vi "Execute.vi"(8 "error in (no error)":errorcluster, 9 "Parameters":map{string, variant}(c390), 10 "Query":string, 11 "Sqlite Database Manager in":refnum<class "Sqlite Database Manager.lvclass">) -> (0 "error out":errorcluster, 3 "Sqlite Database Manager out":refnum<class "Sqlite Database Manager.lvclass">)   [LabVIEW 2019, in "HierDAL Library.lvlib" / "Database.lvlib" / "Sqlite Database Manager.lvclass"]
uses:
  Sqlite Database Manager.lvclass
  Sqlite Database Manager.lvclass/Sqlite Database Manager.ctl
  System.Data.SQLite
  <vilib>/Utility/Data Type/NI_Data Type.lvlib
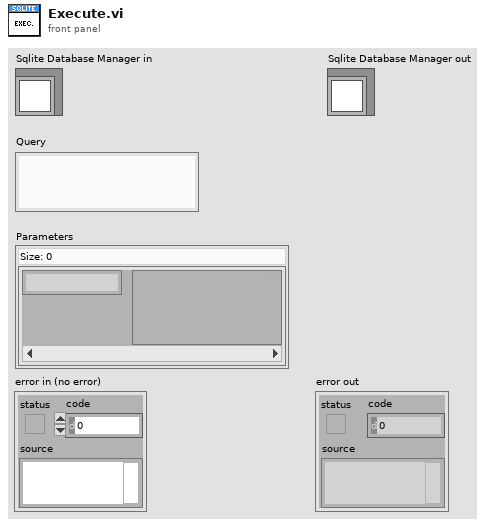
[diagram p1: front panel]
types:
  T1 = typedef "NI_Data Type.lvlib/Data Type.ctl" = enum8{"Invalid Type", "Void", "I8", "I16", "I32", "I64", "U8", "U16", "U32", "U64", "Single Float", "Double Float", "Extended Float", "Single Complex", "Double Complex", "Extended Complex", "Enum U8", "Enum U16", "Enum U32", "Enum U64", "Single Float With Unit", "Double Float With Unit", "Extended Float With Unit", "Single Complex with Unit", "Double Complex with Unit", "Extended Complex with Unit", "Boolean", "String", "Path", "Picture", "Tag", "Array", "Cluster", "Variant", "LV Variant", "Waveform", "Timestamp", "Digital Waveform", "Digital Data", "ExpressData", "Refnum", "External Data", "VI", "Poly VI", "LabVIEW Class Instance", "Fixed Point", "Set Collection", "Map Collection"}
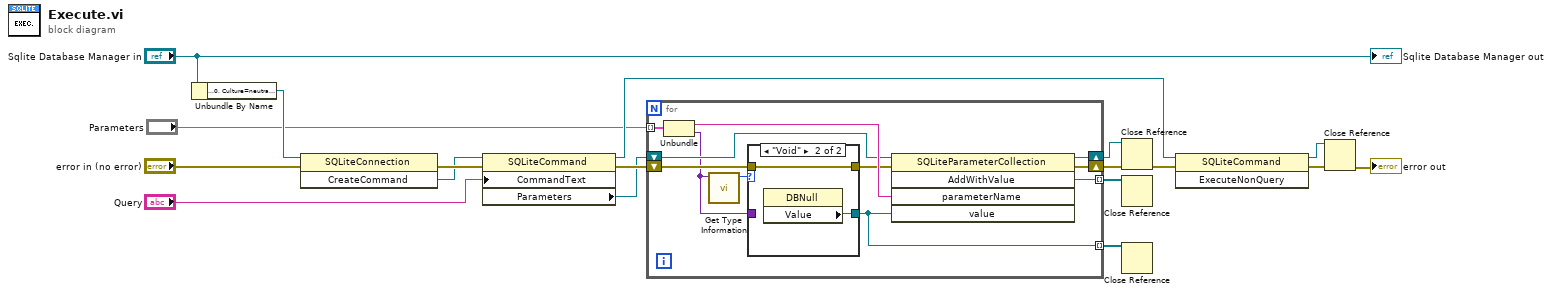
[diagram p0: block diagram]
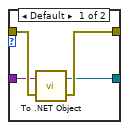
[diagram p2: hidden frame]
diagram:
  n1 = Unbundle By Name("Sqlite Database Manager in") -> ("Connection"=w15:refnum<k24>)
  n2 = invoke class="SQLiteConnection" method="CreateCommand"(reference=w15, error in="error in (no error)") -> (error out=w14:errorcluster, "CreateCommand"=w13:refnum<k24>)  [unwired: 1 in, 1 out]
  n3 = property class="SQLiteCommand"(reference=w13, error in=w14, "CommandText"="Query") -> (reference out=w18:refnum<k24>, error out=w17:errorcluster, "Parameters"=w11:refnum<k24>)
  n4 = for {
    shift-right: [w27] -> w2
    shift-left: w11 -> [w20]
    tunnel: "Parameters" -> [w29] mode=indexing
    shift-right: [w28] -> w3
    shift-left: w17 -> [w22]
    tunnel: [w26] -> w8 mode=indexing
    tunnel: [w25] -> w9 mode=indexing
    n5 = Unbundle(w29) -> ("Parameter"=w24:string, "Value"=w19:variant)
    n6 = call <vilib>:"Get Type Information.vi"("variant"=w19) -> ("type"=w23:T1)  [unwired: 6 in, 4 out]
    n7 = case shown="\"Void\"" w23 {
      tunnel: [w31 w34] -> w25
      tunnel: w22 -> [w33 w35]
      tunnel: [w32 w35] -> w21
      tunnel: w19 -> [w30 _]
      frame Default {
        n8 = call <vilib>:"To .NET Object.vi"("error in (no error)"=w33, "anything"=w30) -> ("error out"=w32:errorcluster, ".NET object"=w31:refnum<k24>)
      }
      frame "Void" {
        n9 = property class="DBNull"() -> ("Value"=w34:refnum<k24>)  [unwired: 2 in, 2 out]
      }
    }
    n10 = invoke class="SQLiteParameterCollection" method="AddWithValue"(reference=w20, error in=w21, "parameterName"=w24, "value"=w25) -> (reference out=w27:refnum<k24>, error out=w28:errorcluster, "AddWithValue"=w26:refnum<k24>)  [unwired: 1 in, 2 out]
  }
  n11 = Close Reference(reference=w2, error in (no error)=w3) -> (error out=w1:errorcluster)
  n12 = Close Reference(reference=w8) -> ()  [unwired: 1 in, 1 out]
  n13 = Close Reference(reference=w9) -> ()  [unwired: 1 in, 1 out]
  n14 = invoke class="SQLiteCommand" method="ExecuteNonQuery"(reference=w18, error in=w1) -> (reference out=w4:refnum<k24>, error out=w6:errorcluster)  [unwired: 1 in, 1 out]
  n15 = Close Reference(reference=w4, error in (no error)=w6) -> (error out=→"error out":errorcluster)
  "Sqlite Database Manager out" <- "Sqlite Database Manager in"
